vi "UI_AutoRefresh.vi"(7 "Sourcer name":string, 8 "error in (no error)":errorcluster, 9 "Parameters (Tipstrips,Captions,All)":T2={"Write TipStrips with details (T)"=TRUE, "Write Captions with UserLabels (T)"=TRUE, "Mode (ind only)"=enum."All", "Enable nested stream (T)"=TRUE}, 10 "Data chunk":T1(array[cluster]), 11 "UI_Actor in":refnum<class "UI_Actor.lvclass">) -> (0 "error out":errorcluster, 3 "UI_Actor out":refnum<class "UI_Actor.lvclass">)   [LabVIEW 2020, in "UI_Actor.lvlib" / "UI_Actor.lvclass"]
uses:
  UI_Actor.lvclass
  ctl_AR_Parameters.ctl
  ctl_AR_Mode.ctl
  support/Databox.lvlibp/TypesTools/Config/Config.lvclass
  support/Databox.lvlibp/TypesTools/Data/Data.lvclass
  support/Databox.lvlibp/TypesTools/Config/Read System Label.vi
  support/Databox.lvlibp
  support/Databox.lvlibp/Databox/Databox.lvclass
  support/Databox.lvlibp/Databox_unsealed/Databox_unsealed.lvclass
  D:/Projets/STEP AT/UI Actor/support/Databox.lvlibp/Databox/Databox.lvclass
  D:/Projets/STEP AT/UI Actor/support/Actor Framework.lvlibp/1abvi3w/vi.lib/ActorFramework/Actor/Actor.lvclass
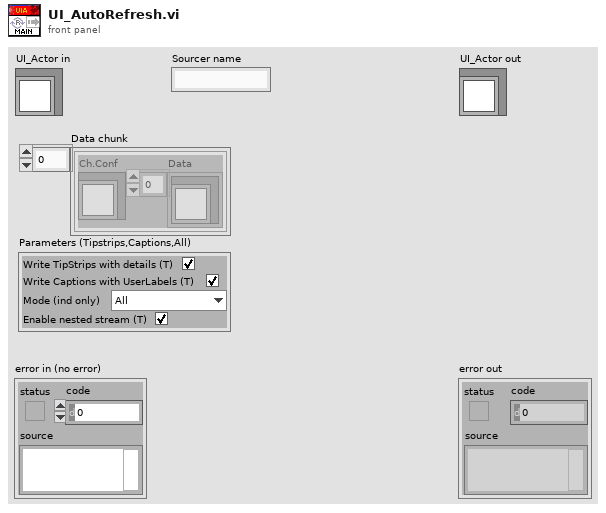
[diagram p1: front panel]
types:
  T1 = cluster{"Ch.Conf":refnum<class "Config.lvclass">, "Data":refnum<class "Data.lvclass">[]}[]
  T2 = typedef "UI_Actor.lvlib/UI_Actor.lvclass/ctl_AR_Parameters.ctl" = cluster{"Write TipStrips with details (T)":bool, "Write Captions with UserLabels (T)":bool, "Mode (ind only)":T3, "Enable nested stream (T)":bool}
  T3 = typedef "UI_Actor.lvlib/UI_Actor.lvclass/ctl_AR_Mode.ctl" = enum16{"Controls only", "Indicators only", "All"}
  T4 = cluster{"Node":string, "Data":refnum<class "Data.lvclass">[]}
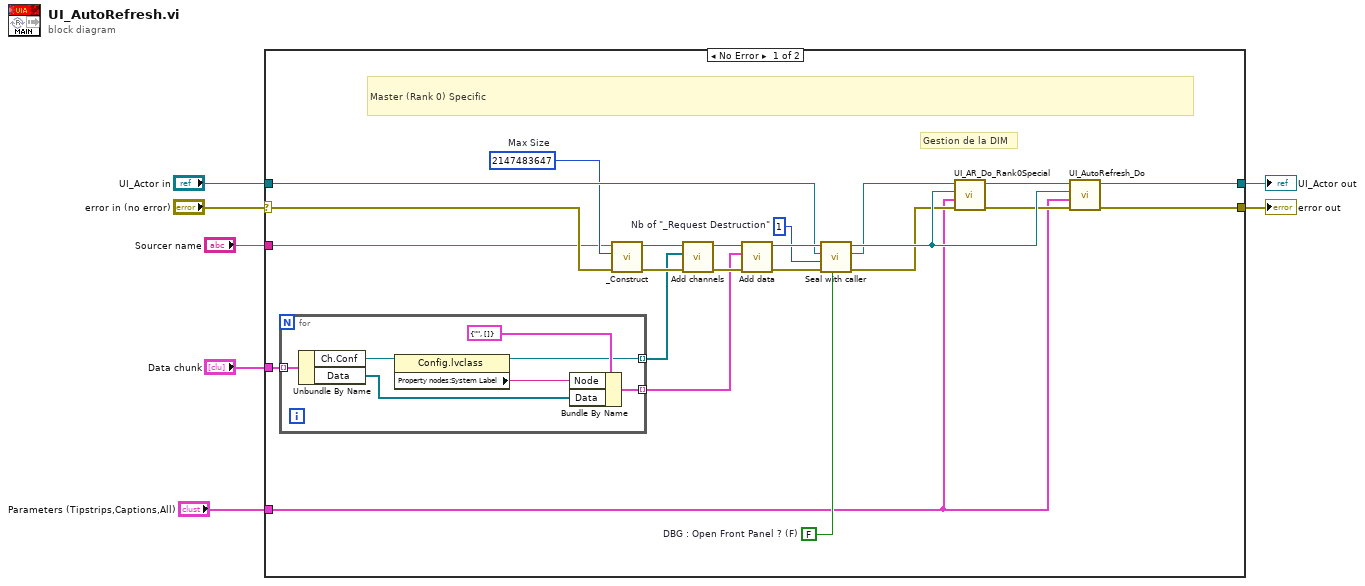
[diagram p0: block diagram]
diagram:
  n1 = case shown="No Error" "error in (no error)" {
    selector: "error in (no error)" -> [w17 w39]
    tunnel: [w18 w39] -> w6
    tunnel: [w19 w38] -> w4
    tunnel: "UI_Actor in" -> [w22 w38]
    tunnel: "Parameters (Tipstrips,Captions,All)" -> [w9 _]
    tunnel: "Data chunk" -> [w24 _]
    tunnel: "Sourcer name" -> [w8 _]
    frame No Error {
      w15 = FALSE  # DBG : Open Front Panel ? (F)
      w16 = 2147483647  # Max Size
      w20 = 1  # Nb of "_Request Destruction"
      # "Gestion de la DIM"
      # "Master (Rank 0) Specific"
      n2 = for {
        tunnel: w24 -> [w37] mode=indexing
        tunnel: [w32] -> w23 mode=indexing
        tunnel: [w34] -> w21 mode=indexing
        n3 = Unbundle By Name(w37) -> ("Ch.Conf"=w36:refnum<class "Config.lvclass">, "Data"=w33:refnum<class "Data.lvclass">[])
        n4 = property class="Config.lvclass"(reference=w36) -> (reference out=w32:refnum<class "Config.lvclass">, "Property nodes:System Label"=w31:string)  [unwired: 1 in, 1 out]
        n5 = Bundle By Name(cluster=T4 {"Node"="", "Data"=[]}, "Node"=w31, "Data"=w33) -> (w34:T4)
      }
      n6 = call "_Construct.vi"("error in (no error)"=w17, "Max Size"=w16, "Builder name"=w8) -> ("error out"=w26:errorcluster, "Databox_unsealed out"=w25:refnum<class "Databox_unsealed.lvclass">)  [unwired: 7 in]
      n7 = call "Add channels.vi"("error in (no error)"=w26, "Channels configs"=w23, "Databox in"=w25) -> ("error out"=w28:errorcluster, "Databox out"=w27:refnum<class "Databox_unsealed.lvclass">)  [unwired: 7 in]
      n8 = call "Add data.vi"("error in (no error)"=w28, "Nodes' Data"=w21, "Databox in"=w27) -> ("error out"=w29:errorcluster, "Databox out"=w30:refnum<class "Databox_unsealed.lvclass">)  [unwired: 7 in]
      n9 = call "Seal with caller.vi"("DBG : Open Front Panel ? (F)"=w15, "error in (no error)"=w29, "Nb of \"_Request Destruction\""=w20, "Caller Actor in"=w22, "Databox_unsealed in"=w30) -> ("error out"=w11:errorcluster, "Caller Actor out"=w13:refnum<class "UI_Actor.lvclass">, "Databox_sealed"=w14:refnum<class "Databox_sealed.lvclass">)  [unwired: 4 in]
      n10 = call "UI_AR_Do_Rank0Special.vi"("error in (no error)"=w11, "Parameters"=w9, "Databox_sealed"=w14, "UI_Actor in"=w13) -> ("error out"=w10:errorcluster, "UI_Actor out"=w12:refnum<class "UI_Actor.lvclass">)  [unwired: 6 in]
      n11 = call-dynamic "UI_AutoRefresh_Do.vi"("error in (no error)"=w10, "Parameters"=w9, "Databox_sealed"=w14, "UI_Actor in"=w12) -> ("error out"=w18:errorcluster, "UI_Actor out"=w19:refnum<class "UI_Actor.lvclass">)  [unwired: 6 in]
    }
    frame Error {
    }
  }
  "error out" <- w6
  "UI_Actor out" <- w4
